vi "Setup image data.vi"() -> (3 "Array":u8[](array[numeric]))   [LabVIEW 2014]
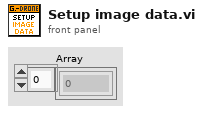
[diagram p1: front panel]
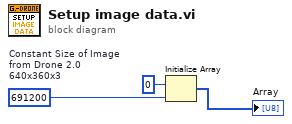
[diagram p0: block diagram]
diagram:
  w2 = 691200  # Constant Size of Image from Drone 2.0 640x360x3
  n1 = Initialize Array(u8 0 ("dimension size"), w2) -> (→"Array":u8[])
